vi "Write RtL GUID.vi"(8 "error in (no error)":errorcluster, 10 "RtL GUID":string, 11 "Monkey in":refnum<class "Tamer.lvclass">) -> (0 "error out":errorcluster, 3 "Monkey out":refnum<class "Tamer.lvclass">)   [LabVIEW 2020, in "CIRCUS_uServices.lvlib" / "Tamer.lvlib" / "Tamer.lvclass"]
uses:
  Tamer.lvclass
  Tamer.lvclass/Tamer.ctl
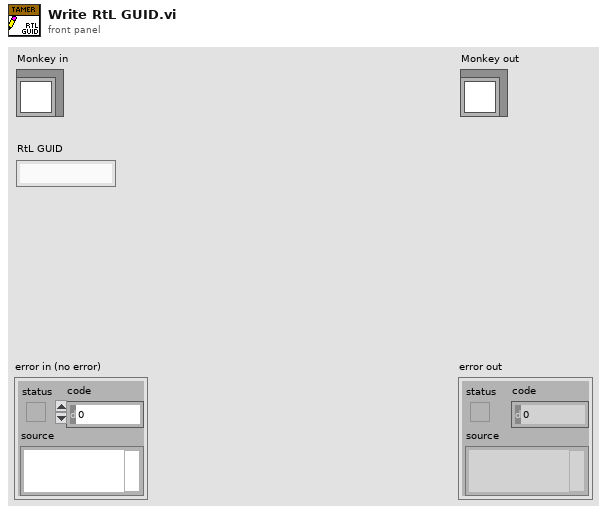
[diagram p1: front panel]
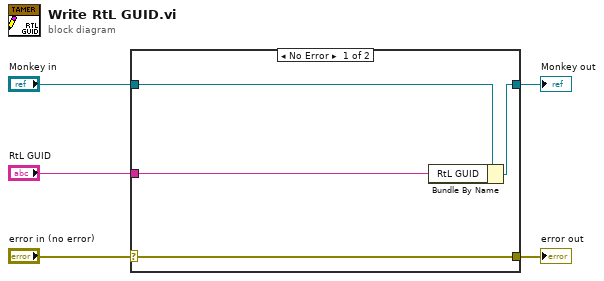
[diagram p0: block diagram]
diagram:
  n1 = case shown="No Error" "error in (no error)" {
    selector: "error in (no error)" -> [w9 w10]
    tunnel: [w9 w10] -> w4
    tunnel: [w7 w11] -> w2
    tunnel: "Monkey in" -> [w8 w11]
    tunnel: "RtL GUID" -> [w6 _]
    frame No Error {
      n2 = Bundle By Name(cluster=w8, "RtL GUID"=w6) -> (w7:refnum<class "Tamer.lvclass">)
    }
    frame Error {
    }
  }
  "error out" <- w4
  "Monkey out" <- w2
